vi "OSA20X_Create.vi"(0 "reference in":refnum<class "OSA.lvclass">, 1 "Graph Intrfrgrm":T3, 2 "Graph Spectrum":T3, 3 "plot zoom step factor":dbl=3.0 format="%.2f", 4 "rel humidity (50%)":dbl=50.0 format="%.2f", 5 "error in (no error)":errorcluster, 6 "spectrometer serial nr":string, 7 "peaks max nr (100)":u32=100, 8 "spectrometer model":string, 9 "spectrometerIdx":u16, 10 "OSA series":T1, 11 "path FTSLV.dll":string="dll\\util", 13 "traces":T2={"nr interferogram (2)"=2, "nr spectrum (10)"=10}) -> (14 "reference":refnum<class "OSA.lvclass">, 19 "error out":errorcluster)   [LabVIEW 2010, in "OSA.lvclass"]
doc: "Creates and initializes a new <B>Thorlabs_OSA_64</B> object.\n\nThis object should be destroyed using a <B>Thorlabs_OSA_64 destructor</B> VI.\n\n[GOOP 1.0]"
uses:
  OSA.lvclass
  private/graph_intensity.ctl
  typeDef/OSA_series.ctl
  action_data.ctl
  typeDef/queue_action.ctl
  typeDef/acq_dataType.ctl
  OSA.lvclass/OSA.ctl
  OSA20X_misc.lvlib
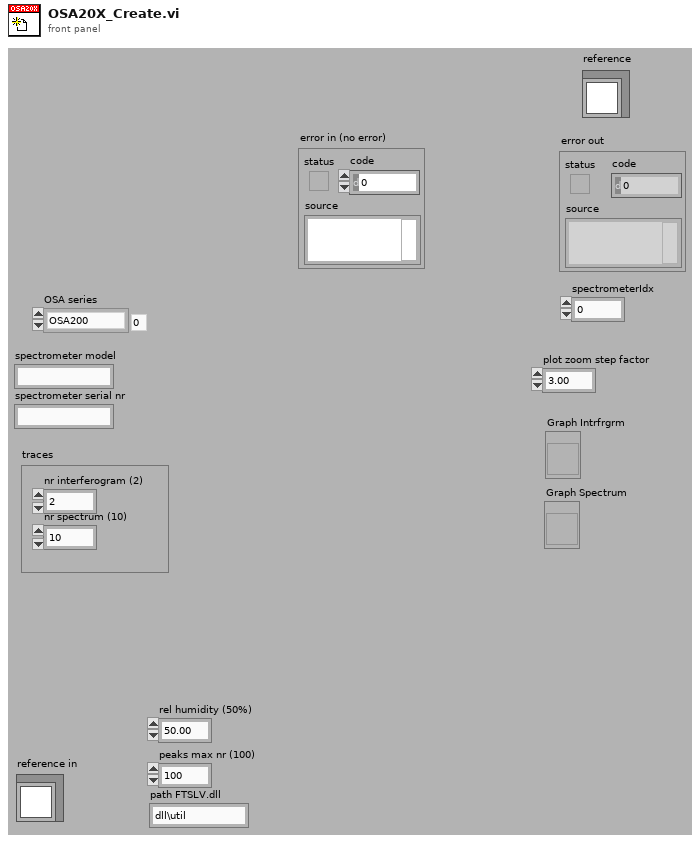
[diagram p1: front panel]
types:
  T1 = typedef "OSA.lvclass/OSA_series.ctl" = enum16{"OSA200", "OSA300", "UNKNOWN"}
  T2 = cluster{"nr interferogram (2)":i32, "nr spectrum (10)":i32}
  T3 = typedef "OSA.lvclass/graph_intensity.ctl" = refnum<vi>
  T4 = typedef "OSA.lvclass/action_data.ctl" = cluster{"action":T5, "skip old":bool, "force immidiate":bool, "par":dbl, "par 2":dbl, "par 3":dbl, "par 4":dbl, "idx":i32, "idx 2":i32, "no duplicate":bool}
  T5 = typedef "OSA.lvclass/queue_action.ctl" = enum16{"none", "stop", "GUI_plotInterferogram", "GUI_plotSpectrum", "GUI_plotInterferogramRescale", "GUI_plotSpectrumRescale", "GUI_plotInterferogramReset", "GUI_plotSpectrumReset", "GUI_plotInterferogramAutoScaleY", "GUI_plotSpectrumAutoScaleY", "GUI_plotInterferogramZoomOut", "GUI_plotSpectrumZoomOut", "GUI_plotInterferogramPane", "GUI_plotSpectrumPane", "GUI_plotInterferogramZoomMouse", "GUI_plotSpectrumZoomMouse", "ENVIRONMENT temperature", "ENVIRONMENT pressure", "MODE_resolution set", "MODE_resolution get", "MODE_sensitivity set", "MODE_sensitivity get", "MODE_PDTemperature set", "MODE_PDTemperature get", "REBOOT/RESET firmware", "ACQASYNC_acquireSingleSpectrum", "ACQASYNC_continuous start", "ACQASYNC_continuous stop\n", "ACQASYNC_get last interferogram", "ACQASYNC_get last spectrum", "ACQASYNC_get last waveNr", "ACQOPT_interferogram smoothing set", "ACQOPT_interferogram smoothing get", "ACQOPT_spectrum smoothing set", "ACQOPT_spectrum smoothing get", "ACQOPT_apodisation type set", "ACQOPT_apodisation type get", "ACQOPT_phase correction type set", "ACQOPT_phase correction type get", "ACQOPT_acqIntervall_set", "ACQOPT_acqIntervall_get", "ACQOPT_average spectrum set", "ACQOPT_average spectrum get", "ACQOPT_rolling average set", "ACQOPT_rolling average get", "ACQOPT_zero fill factor set", "ACQOPT_zero fill factor get", "ACQOPT_cycle counting set", "ACQOPT_cycle counting get", "ACQOPT_air measure option set", "ACQOPT_air measure option get", "ACQOPT_gainLevel auto get", "ACQOPT_gainLevel auto set", "ACQOPT_gainLevel get", "ACQOPT_gainLevel set", "ACQOPT_getAll", "INSTRUMENT_PROPERTY_range_WaveNr_min", "INSTRUMENT_PROPERTY_range_WaveNr_max", "INSTRUMENT_PROPERTY_reference_wavelength_cm^-1", "INSTRUMENT_PROPERTY_samplesPerRefPeriod", "INSTRUMENT_PROPERTY_resolution_waveNrPercm", "INSTRUMENT_PROPERTY_availableGainLevels", "INSTRUMENT_PROPERTY_status", "CONVERT", "ANALYSE_POWER", "ANALYSE_PEAKS", "ANALYSE_WAVELENGTH", "ANALYSE_SPECTRUM", "ANALYSE_INTERFEROGRAM", "ANALYSE_COHERENCE_LENGTH", "MATH", "MATH_power", "MATH_peaks", "FILE", "miscellaneous"}
  T6 = cluster{"idx":u32, "broadBand":bool, "monoChromatic":bool, "peakToPeakSignal":dbl, "peakToPeakPos":dbl}
  T7 = typedef "OSA.lvclass/acq_dataType.ctl" = enum16{"none", "interferogram", "spectrum"}
  T8 = typedef "Semaphore RefNum" = refnum<k1>
  T9 = typedef "OSA.lvclass/ObjectAttributes.ctl" = cluster{"Stop":bool, "dataType":T7, "spectrometerIdx":u16, "buffer size interferogram":i32, "interferogram":cluster{"new":bool, "plot_x_ min":sgl, "plot_x_max":sgl, "plot_y_min":sgl, "plot_y_max":sgl, "Graph Intrfrgrm":T3, "timeStamp":u32, "signal (%)":dbl, "traces":cluster{"idx":u32, "broadBand":bool, "monoChromatic":bool, "peakToPeakSignal":dbl, "peakToPeakPos":dbl}[], "traces idx last":i32}, "spectrum":cluster{"new":bool, "plot_x_min":sgl, "plot_x_max":sgl, "plot_unit_x":T10, "plot_unit_y":T11, "plot_y_min":sgl, "plot_y_max":sgl, "Graph Spectrum":T3, "timeStamp":u32, "X_VAL_OPTIONS":enum16{"MIN_MAX", "ARRAY"}, "traces":cluster{"idx":u32}[], "traces idx last":i32}, "Thorlabs_OSA_64.lvclass:queue_action.ctlqueue ref":refnum<queue>, "action":T5, "plot zoom step":dbl, "buffer semaphore":T8, "acq stopped":bool, "dataType active":T7, "temperature (degr C)":sgl, "pressure (hPa)":sgl, "rel humidity (%)":sgl, "settings":cluster{"resolution":T12, "sensitivity":T13, "Average":bool, "average nr":u32, "apodisation":T14, "acq delay (ms)":u32, "airMesure":T15, "wmtr on":bool, "intfgrm_smooth_width":u16, "intfgrm_smooth_nrOfPasses":u16, "intfgrm_smooth":T16, "phaseCorrection":T17, "zeroFill":u8, "spectr_smooth":T16, "spectr_smooth_width":u16, "spectr_smooth_nrOfPasses":u16, "resolution (/cm)":sgl, "REF wavelength, (nm)":dbl, "gain_idx":u16, "gainAuto":bool, "gain_relative":dbl, "PD sensitivity mode":T18, "PD senseMode implemented":bool, "SensorTemperature implemented":bool, "SensorPressure implemented":bool, "SensorHumidity implemented":bool}, "peaks position":sgl[], "peaks width":sgl[], "peaks height":sgl[], "peaks max nr":u32, "peaks latest nr":i32, "peaks new":bool, "power":dbl, "power new":bool, "path":string, "wavelength (WNr)":dbl, "wavelength new":bool, "buffer size spectrum":i32, "status":string, "VI reference":refnum<vi>, "funcPointer":u64, "libraryPointer":u64, "singleAcquisition":bool, "coherenceLength (cm)":dbl, "coherenceLength new":bool, "spectrometer model":string, "spectrometer serial nr":string, "peaks thld left":sgl[], "peaks thld right":sgl[], "coherenceLength error (cm)":dbl, "ADC bits":u16, "peaks position centroid":sgl[], "peaks height centroid":sgl[], "OSA series":T1, "channel index spectrum":u16, "spectrometer rangeLow, (/cm)":dbl, "spectrometer rangeHigh, (/cm)":dbl, "channel index interferogram":u16}
  T10 = typedef "OSA.lvclass/spectrum_x_unit.ctl" = enum16{"wavenr/cm", "THz", "eV", "nm_air", "nm_vac"}
  T11 = typedef "OSA.lvclass/y_unit.ctl" = enum16{"ADC counts", "dBm pwr absolute", "dBm pwr density", "mW pwr absolute", "mW pwr density"}
  T12 = typedef "OSA.lvclass/resolution.ctl" = enum16{"low", "high"}
  T13 = typedef "OSA.lvclass/sensitivityMode.ctl" = enum16{"low", "low medium", "high medium", "high"}
  T14 = typedef "OSA.lvclass/apodisation.ctl" = enum16{"NONE", "NORTON_BEER_WEAK", "NORTON_BEER_MEDIUM", "NORTON_BEER_STRONG", "TRIANGULAR", "COSINE", "HANN", "HAMMING", "BLACKMANHARRIS3", "BLACKMANHARRIS4", "GAUSSIAN"}
  T15 = typedef "OSA.lvclass/airMeasure.ctl" = enum16{"TEMPERATURE", "PRESSURE"}
  T16 = typedef "OSA.lvclass/smoothing.ctl" = enum16{"NONE", "BINOMIAL", "SAVITSKY_GOLAY", "FOURIER", "MOVING_AVERAGE", "GAUSSIAN"}
  T17 = typedef "OSA.lvclass/phaseCorrection.ctl" = enum16{"NONE", "MERTZ", "FORMAN", "MERTZ_FILE", "FORMAN_FILE", "FUTURE COMP."}
  T18 = typedef "OSA.lvclass/PDTemperatureMode.ctl" = enum16{"cool: better sensitivity/noise floor", "warm: extended wl range"}
  T19 = cluster{"idx":u32, "broadBand":bool, "monoChromatic":bool, "peakToPeakSignal":dbl, "peakToPeakPos":dbl}[]
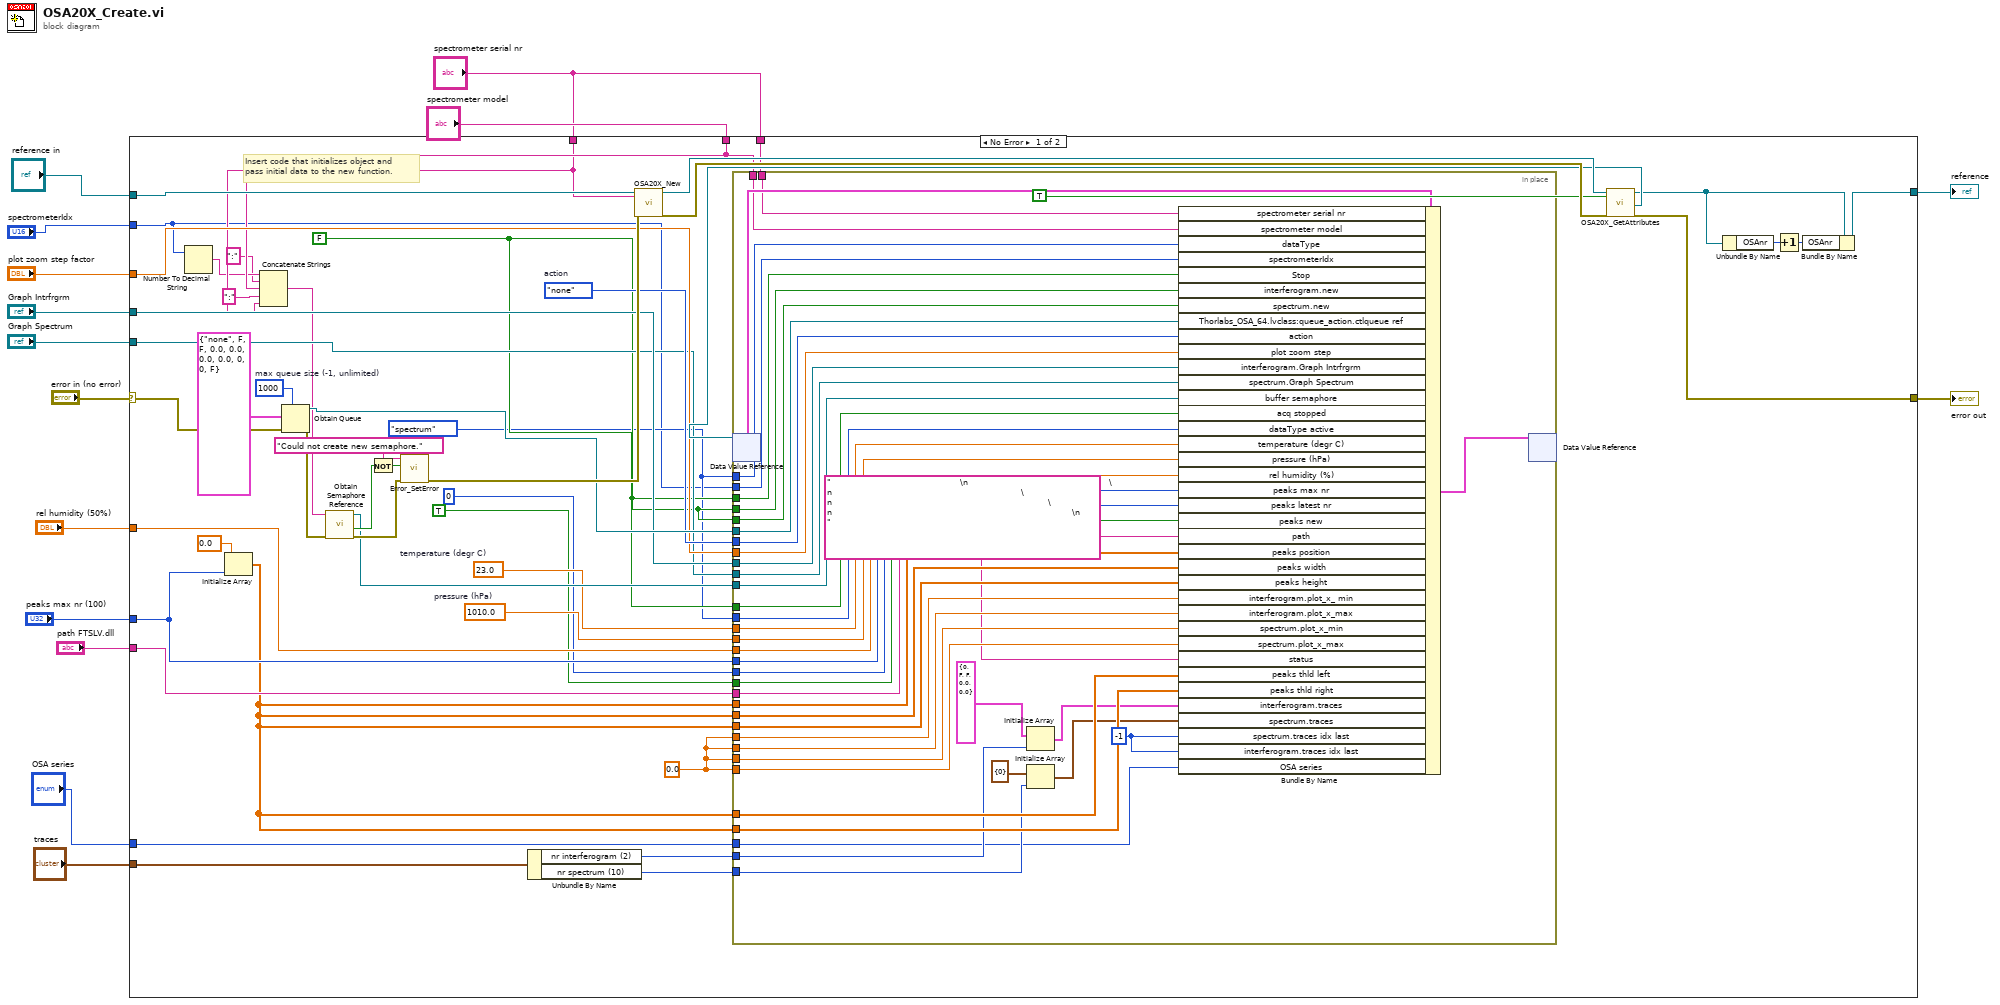
[diagram p0: block diagram]
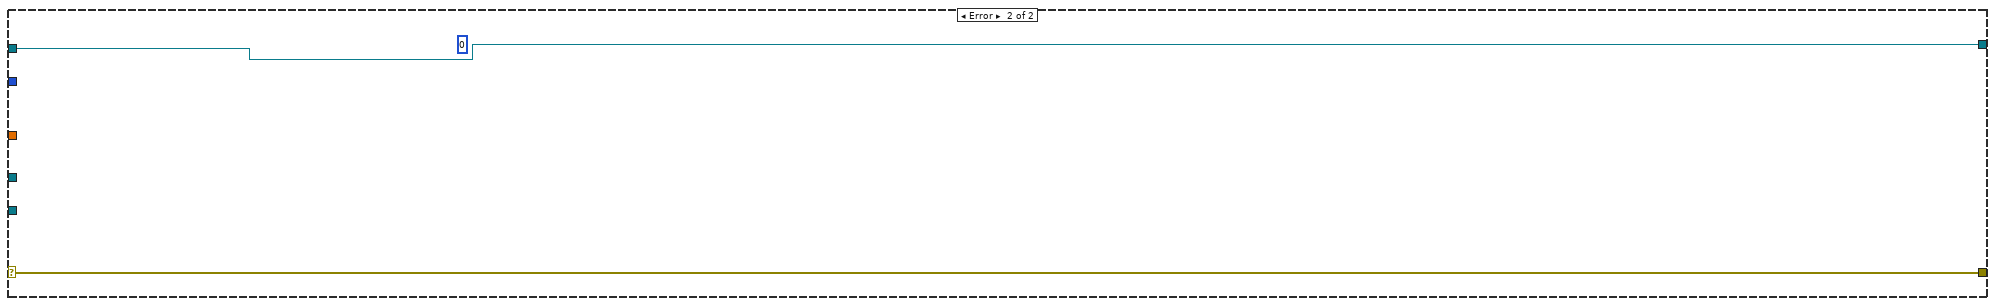
[diagram p2: hidden frame]
diagram:
  n1 = case shown="No Error" "error in (no error)" {
    selector: "error in (no error)" -> [w64 w108]
    tunnel: [w52 w108] -> w15
    tunnel: [w30 w107] -> w14
    tunnel: "spectrometerIdx" -> [w22 _]
    tunnel: "Graph Intrfrgrm" -> [w44 _]
    tunnel: "Graph Spectrum" -> [w43 _]
    tunnel: "plot zoom step factor" -> [w45 _]
    tunnel: "rel humidity (50%)" -> [w37 _]
    tunnel: "peaks max nr (100)" -> [w36 _]
    tunnel: "path FTSLV.dll" -> [w33 _]
    tunnel: "reference in" -> [w51 w107]
    tunnel: "spectrometer serial nr" -> [w48 _]
    tunnel: "spectrometer model" -> [w26 _]
    tunnel: "spectrometer serial nr" -> [w24 _]
    tunnel: "traces" -> [w19 _]
    tunnel: "OSA series" -> [w16 _]
    frame No Error {
      w32 = sgl 0.0 ("interferogram.plot_x_ min")
      w38 = sgl 1010.0  # pressure (hPa)
      w39 = sgl 23.0  # temperature (degr C)
      w40 = acq_dataType."spectrum" ("dataType active")
      w46 = queue_action."none"  # action
      w62 = 1000  # max queue size (-1, unlimited)
      w41 = FALSE ("Stop")
      # "Insert code that initializes object and\npass initial data to the new function."
      n2 = Number To Decimal String(number=w22) -> (decimal integer string=w21:string)  [unwired: 1 in]
      n3 = Initialize Array(sgl 0.0, w36) -> (w31:sgl[])
      n4 = Concatenate Strings(w21, ":" ("string"), w26, ":" ("string"), w24) -> (w23:string)
      n5 = Obtain Queue(max queue size (-1, unlimited)=w62, element data type=T4 {"action"=enum."none", "skip old"=FALSE, "force immidiate"=FALSE, "par"=0.0, "par 2"=0.0, "par 3"=0.0, "par 4"=0.0, "idx"=0, "idx 2"=0, "no duplicate"=FALSE} ("element"), error in (no error)=w64) -> (queue out=w47:refnum<queue>, error out=w57:errorcluster)  [unwired: 2 in, 1 out]
      n6 = call <vilib>:"Obtain Semaphore Reference.vi"("error in (no error)"=w57, "name (unnamed)"=w23) -> ("error out"=w56:errorcluster, "created new"=w60:bool, "semaphore"=w42:T8)  [unwired: 3 in]
      n7 = Not(x=w60) -> (.not. x?=w59:bool)
      n8 = call "Error_SetError.vi"("error in"=w56, "status (true)"=w59, "source(\"\")"="Could not create new semaphore." ("source(\"\")")) -> ("error out"=w61:errorcluster)  [unwired: 4 in]
      n9 = Unbundle By Name(w19) -> ("nr interferogram (2)"=w18:i32, "nr spectrum (10)"=w17:i32)
      n10 = call "OSA20X_New.vi"("reference in"=w51, "Object name"=w24, "error in (no error)"=w61) -> ("reference out"=w54:refnum<class "OSA.lvclass">, "error out"=w53:errorcluster)  [unwired: 13 in, 2 out]
      n11 = call "OSA20X_GetAttributes.vi"("reference in"=w54, "OnlyGetDvrReference(False)"=TRUE, "error in (no error)"=w53) -> ("reference out"=w29:refnum<class "OSA.lvclass">, "DataRef"=w49:refnum<data-value>, "error out"=w52:errorcluster)  [unwired: 13 in, 1 out]
      n12 = in-place {
        in-place-border: w48 -> [w105]
        in-place-border: w26 -> [w104]
        in-place-border: w40 -> [w103]
        in-place-border: w22 -> [w102]
        in-place-border: w41 -> [w101]
        in-place-border: w41 -> [w100]
        in-place-border: w41 -> [w99]
        in-place-border: w47 -> [w98]
        in-place-border: w46 -> [w97]
        in-place-border: w45 -> [w96]
        in-place-border: w44 -> [w95]
        in-place-border: w43 -> [w94]
        in-place-border: w42 -> [w93]
        in-place-border: w41 -> [w92]
        in-place-border: w40 -> [w91]
        in-place-border: w39 -> [w90]
        in-place-border: w38 -> [w89]
        in-place-border: w37 -> [w88]
        in-place-border: w36 -> [w87]
        in-place-border: 0 ("peaks latest nr") -> [w86]
        in-place-border: TRUE ("peaks new") -> [w85]
        in-place-border: w33 -> [w84]
        in-place-border: w31 -> [w83]
        in-place-border: w31 -> [w82]
        in-place-border: w31 -> [w81]
        in-place-border: w32 -> [w80]
        in-place-border: w32 -> [w79]
        in-place-border: w32 -> [w78]
        in-place-border: w32 -> [w77]
        in-place-border: w31 -> [w74]
        in-place-border: w31 -> [w73]
        in-place-border: w18 -> [w70]
        in-place-border: w17 -> [w69]
        in-place-border: w16 -> [w65]
        w68 = -1 ("spectrum.traces idx last")
        n13 = in-place-dvr #1(w49) -> (w106:T9)  [unwired: 1 out]
        n14 = Initialize Array(T6 {"idx"=0, "broadBand"=FALSE, "monoChromatic"=FALSE, "peakToPeakSignal"=0.0, "peakToPeakPos"=0.0} ("Cluster"), w70) -> (w66:T19)
        n15 = Initialize Array(cluster{"idx":u64} {"idx"=0} ("Cluster"), w69) -> (w71:cluster{"idx":u64}[])
        n16 = Bundle By Name(cluster=w106, "spectrometer serial nr"=w105, "spectrometer model"=w104, "dataType"=w103, "spectrometerIdx"=w102, "Stop"=w101, "interferogram.new"=w100, "spectrum.new"=w99, "Thorlabs_OSA_64.lvclass:queue_action.ctlqueue ref"=w98, "action"=w97, "plot zoom step"=w96, "interferogram.Graph Intrfrgrm"=w95, "spectrum.Graph Spectrum"=w94, "buffer semaphore"=w93, "acq stopped"=w92, "dataType active"=w91, "temperature (degr C)"=w90, "pressure (hPa)"=w89, "rel humidity (%)"=w88, "peaks max nr"=w87, "peaks latest nr"=w86, "peaks new"=w85, "path"=w84, "peaks position"=w83, "peaks width"=w82, "peaks height"=w81, "interferogram.plot_x_ min"=w80, "interferogram.plot_x_max"=w79, "spectrum.plot_x_min"=w78, "spectrum.plot_x_max"=w77, "status"="                                           \n                                               \n                                                               \n                                                                        \n                                                                                \n                                                                                                   ", "peaks thld left"=w74, "peaks thld right"=w73, "interferogram.traces"=w66, "spectrum.traces"=w71, "spectrum.traces idx last"=w68, "interferogram.traces idx last"=w68, "OSA series"=w65) -> (w76:T9)
        n17 = in-place-dvr #1(w76) -> ()  [unwired: 2 out]
      }
      n18 = Unbundle By Name(w29) -> ("OSAnr"=w28:i32)
      n19 = Increment(x=w28) -> (x+1=w27:i32)
      n20 = Bundle By Name(cluster=w29, "OSAnr"=w27) -> (w30:refnum<class "OSA.lvclass">)
    }
    frame Error {
      (unwired) 0
    }
  }
  "error out" <- w15
  "reference" <- w14
